vi "MS Init.vi"(10 "VISA resource name":refnum<visa-resource-name>="COM13", 11 "VISA Refnum in":refnum<visa-resource-name>="COM12") -> (0 "error out":errorcluster, 2 "VISA Refnum out 2":refnum<visa-resource-name>, 3 "VISA Refnum out":refnum<visa-resource-name>)   [LabVIEW 2012]
uses:
  <vilib>/Instr/_visa.llb/VISA Configure Serial Port (Instr).vi
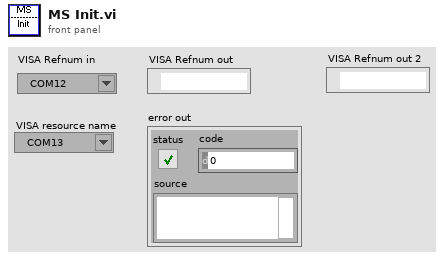
[diagram p1: front panel]
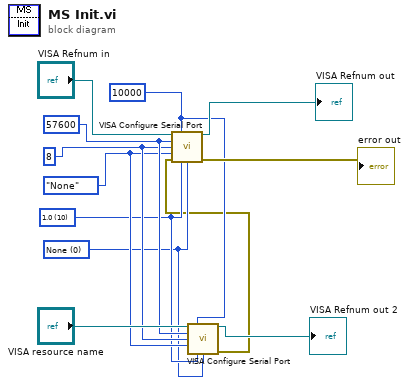
[diagram p0: block diagram]
diagram:
  w8 = u32 10000 ("timeout (10sec)")
  w3 = u16 0 items=["None", "XON/XOFF", "RTS/CTS", "XON/XOFF & RTS/CTS", "DTR/DSR", "XON/XOFF & DTR/DSR"] ("flow control (0:none)")
  w4 = u16 10 items=["1.0"=10, "1.5"=15, "2.0"=20] ("stop bits (10: 1 bit)")
  w5 = enum16{"None", "Odd", "Even", "Mark", "Space"}."None" ("parity (0:none)")
  w6 = u16 8 ("data bits (8)")
  w7 = u32 57600 ("baud rate (9600)")
  n1 = call-poly "VISA Configure Serial Port"("VISA resource name"="VISA resource name", "timeout (10sec)"=w8, "baud rate (9600)"=w7, "data bits (8)"=w6, "parity (0:none)"=w5, "stop bits (10: 1 bit)"=w4, "flow control (0:none)"=w3) -> ("VISA resource name out"=→"VISA Refnum out 2":refnum<visa-resource-name>, "error out"=w1:errorcluster)  [unwired: 7 in]
  n2 = call-poly "VISA Configure Serial Port"("VISA resource name"="VISA Refnum in", "timeout (10sec)"=w8, "baud rate (9600)"=w7, "data bits (8)"=w6, "parity (0:none)"=w5, "error in (no error)"=w1, "stop bits (10: 1 bit)"=w4, "flow control (0:none)"=w3) -> ("VISA resource name out"=→"VISA Refnum out":refnum<visa-resource-name>, "error out"=→"error out":errorcluster)  [unwired: 6 in]
